vi "stoppen_bij_stopstreep_deel2 (SubVI).vi"(11 "gelezen waardes door reflectiesensor":dbl[](array[numeric])) -> (0 "Boolean":bool)   [LabVIEW 2019]
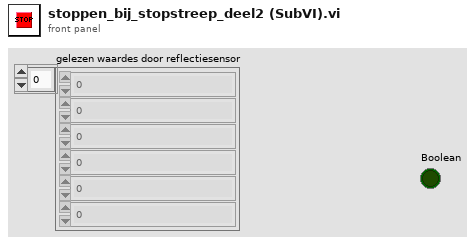
[diagram p1: front panel]
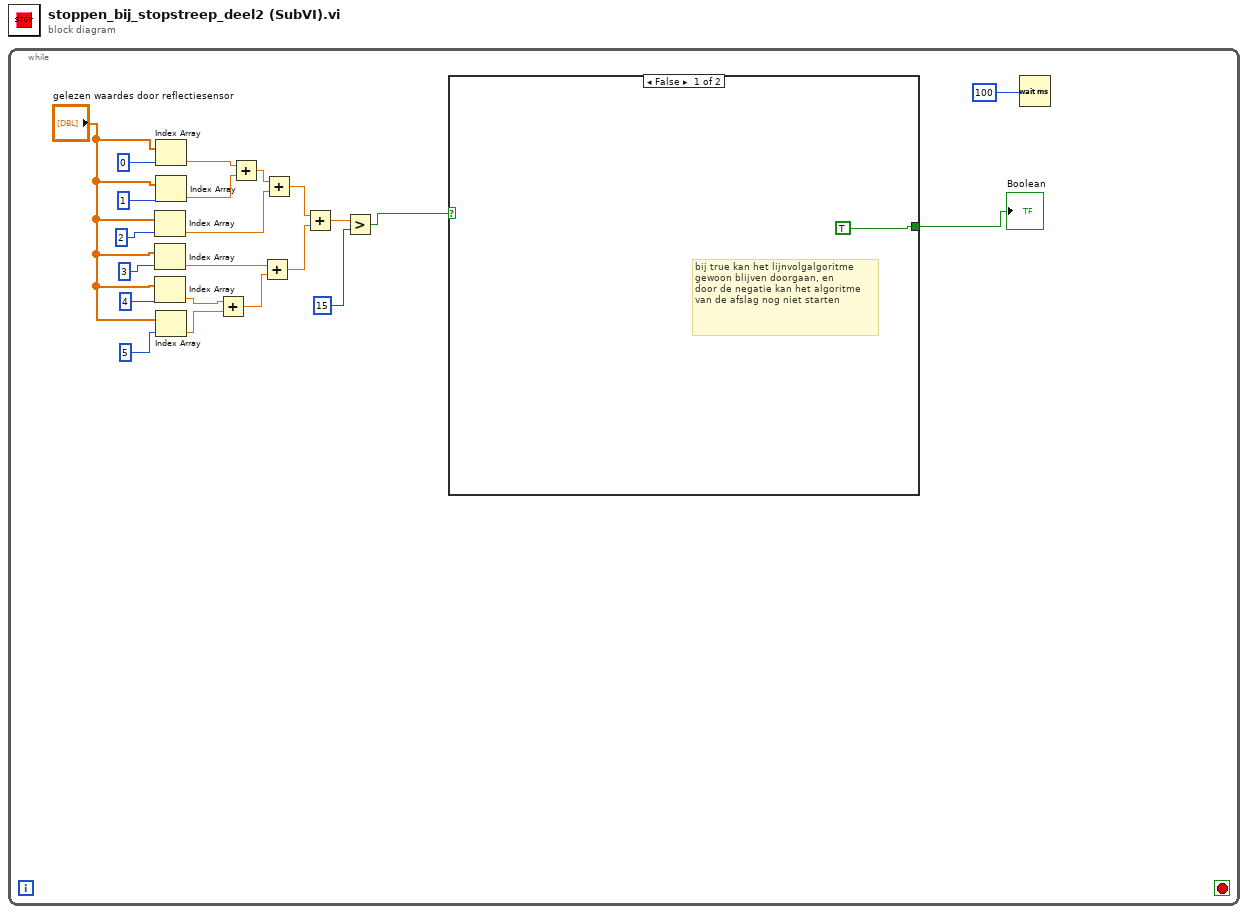
[diagram p0: block diagram]
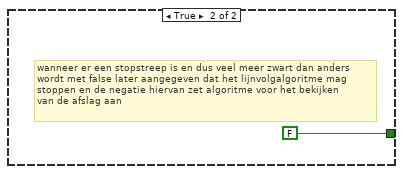
[diagram p2: hidden frame]
diagram:
  n1 = while {
    stop <- _ stop-if-true
    n2 = Index Array(array="gelezen waardes door reflectiesensor", index=2) -> (element=w8:dbl)
    n3 = Index Array(array="gelezen waardes door reflectiesensor", index=3) -> (element=w13:dbl)
    n4 = Index Array(array="gelezen waardes door reflectiesensor", index=4) -> (element=w14:dbl)
    n5 = Index Array(array="gelezen waardes door reflectiesensor", index=0) -> (element=w11:dbl)
    n6 = Index Array(array="gelezen waardes door reflectiesensor", index=1) -> (element=w10:dbl)
    n7 = Index Array(array="gelezen waardes door reflectiesensor", index=5) -> (element=w15:dbl)
    n8 = Add(x=w14, y=w15) -> (x+y=w12:dbl)
    n9 = Add(x=w11, y=w10) -> (x+y=w9:dbl)
    n10 = Add(x=w13, y=w12) -> (x+y=w6:dbl)
    n11 = Add(x=w9, y=w8) -> (x+y=w7:dbl)
    n12 = Add(x=w7, y=w6) -> (x+y=w5:dbl)
    n13 = Greater?(x=w5, y=15) -> (0:w3:bool)
    n14 = case shown="False" w3 {
      tunnel: [TRUE FALSE] -> w2
      frame False {
        # "bij true kan het lijnvolgalgoritme \ngewoon blijven doorgaan, en \ndoor de negatie kan het algoritme \nvan de afslag nog niet starten"
      }
      frame True {
        # "wanneer er een stopstreep is en dus veel meer zwart dan anders \nwordt met false later aangegeven dat het lijnvolgalgoritme mag \nstoppen en de negatie hiervan zet algoritme voor het bekijken \nvan de afslag aan"
      }
    }
    "Boolean" <- w2
    n15 = Wait (ms)(milliseconds to wait=100) -> ()  [unwired: 1 out]
  }
